vi "createChannel.vi"(8 "error in (no error)":errorcluster, 11 "niDAQmxAO in":refnum<class "niDAQmxAO.lvclass">) -> (0 "error out":errorcluster, 3 "niDAQmxAO out":refnum<class "niDAQmxAO.lvclass">)   [LabVIEW 2009, in "Hardware.lvlib" / "Channels.lvlib" / "niDAQmxAO.lvclass"]
uses:
  niDAQmxAO.lvclass
  <vilib>/DAQmx/create/channels.llb/DAQmx Create Channel (AO-Voltage-Basic).vi
  niDAQmxAO.lvclass/niDAQmxAO.ctl
  <vilib>/DAQmx/create/channels.llb/DAQmx Create Channel (AO-Current-Basic).vi
  <vilib>/DAQmx/create/channels.llb/DAQmx Create Channel (AO-FuncGen).vi
  AnalogOutput.lvclass
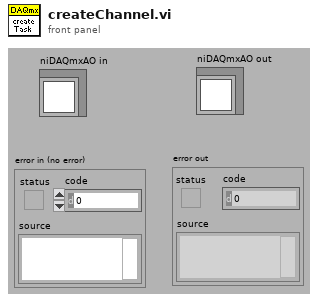
[diagram p1: front panel]
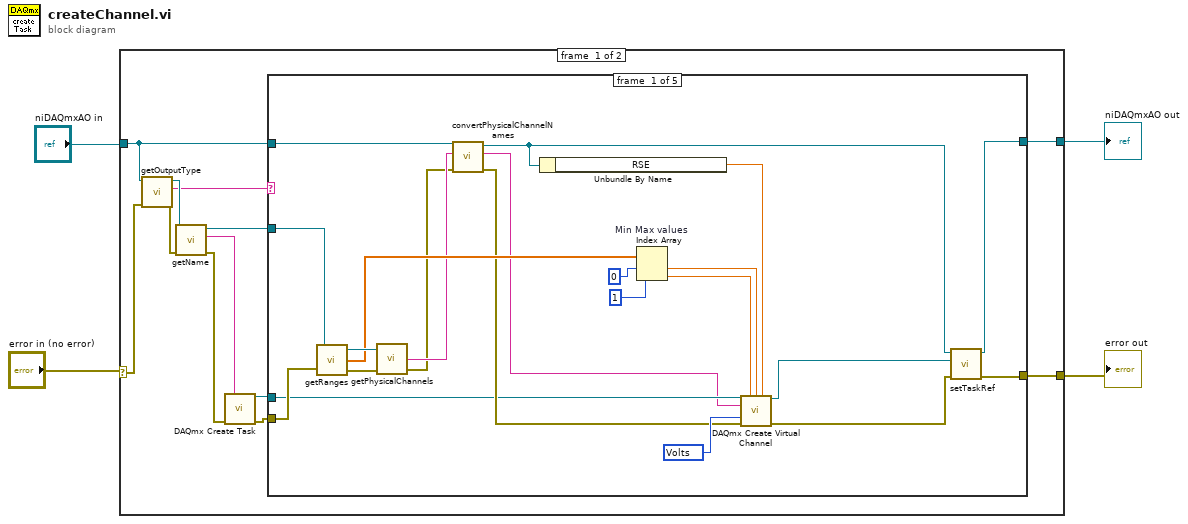
[diagram p0: block diagram]
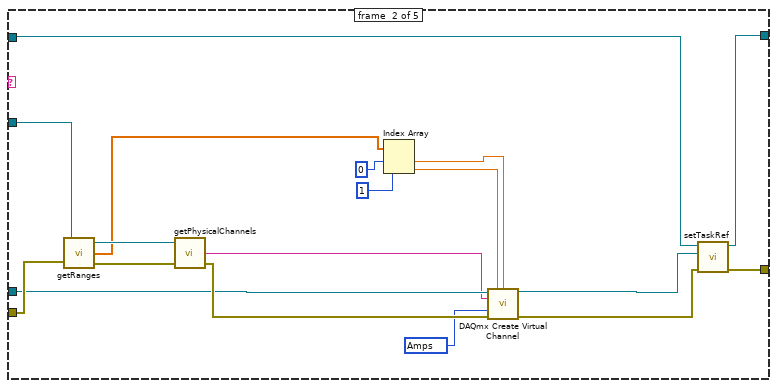
[diagram p2: hidden frame]
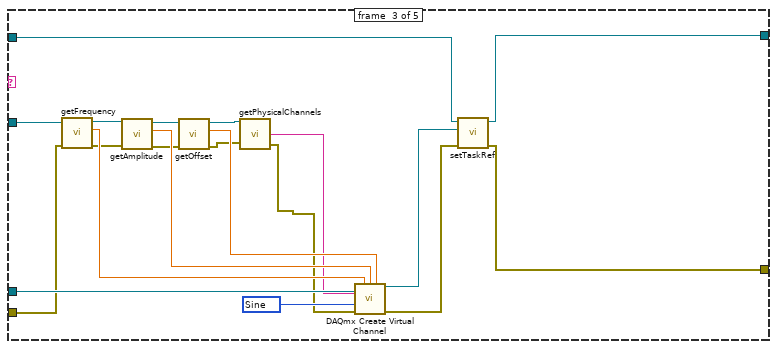
[diagram p3: hidden frame]
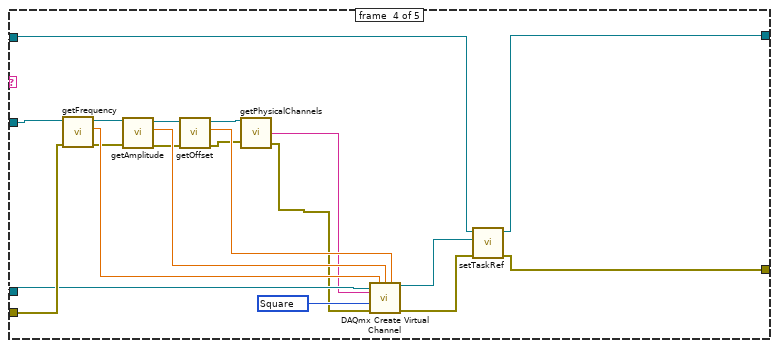
[diagram p4: hidden frame]
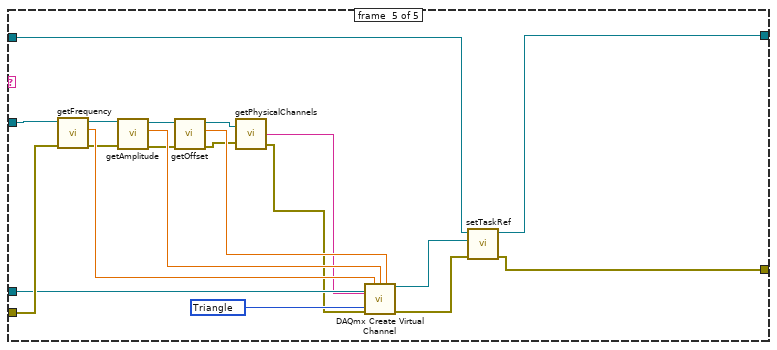
[diagram p5: hidden frame]
diagram:
  n1 = case shown="No Error" "error in (no error)" {
    selector: "error in (no error)" -> [w11 w117]
    tunnel: "niDAQmxAO in" -> [w13 w118]
    tunnel: [w16 w117] -> w2
    tunnel: [w15 w118] -> w1
    frame #0 {
      n2 = call "getOutputType.vi"("error in (no error)"=w11, "AnalogOutput.lvclass in"=w13) -> ("error out"=w10:errorcluster, "Output Type"=w9:string, "AnalogOutput.lvclass out"=w12:refnum<class "niDAQmxAO.lvclass">)  [unwired: 7 in]
      n3 = call "getName.vi"("error in (no error)"=w10, "AnalogOutput.lvclass in"=w12) -> ("error out"=w6:errorcluster, "name"=w5:string, "AnalogOutput.lvclass out"=w14:refnum<class "niDAQmxAO.lvclass">)  [unwired: 7 in]
      n4 = call <vilib>:"DAQmx Create Task.vi"("new task name"=w5, "error in"=w6) -> ("task out"=w8:refnum<k21>, "error out"=w7:errorcluster)  [unwired: 12 in]
      n5 = case shown="\"Voltage\", Default" w9 {
        tunnel: w14 -> [w37 w49 w73 w83 w103]
        tunnel: w8 -> [w18 w47 w62 w81 w101]
        tunnel: w7 -> [w36 w48 w61 w82 w102]
        tunnel: w13 -> [w23 w46 w64 w84 w104]
        tunnel: [w33 w50 w59 w79 w99] -> w16
        tunnel: [w32 w51 w60 w80 w100] -> w15
        frame #0 {
          w25 = u16 10348 items=["Volts"=10348]
          n6 = call "getRanges.vi"("AnalogOutput.lvclass in"=w37, "error in (no error)"=w36) -> ("AnalogOutput.lvclass out"=w31:refnum<class "niDAQmxAO.lvclass">, "Ranges"=w24:dbl[], "error out"=w30:errorcluster)
          n7 = call-dynamic "getPhysicalChannels.vi"("AnalogOutput.lvclass in"=w31, "error in (no error)"=w30) -> ("Physical Channels"=w21:string, "error out"=w20:errorcluster)  [unwired: 1 out]
          n8 = call "convertPhysicalChannelNames.vi"("error in (no error)"=w20, "PhysicalChannels"=w21, "niDAQmxAO.lvclass in"=w23) -> ("error out"=w19:errorcluster, "channel_names"=w17:string, "niDAQmxAO.lvclass out"=w22:refnum<class "niDAQmxAO.lvclass">)  [unwired: 6 in]
          n9 = Unbundle By Name(w22) -> ("RSE"=w38:dbl)
          n10 = Index Array "Min Max values"(array=w24, index #1=0, index #2=1) -> (element #1=w27:dbl, element #2=w26:dbl)
          n11 = call-poly <vilib>:"DAQmx Create Virtual Channel.vi"("task in"=w18, "maximum value"=w26, "minimum value"=w27, "output terminal configuration"=w38, "physical channels"=w17, "units"=w25, "error in"=w19) -> ("task out"=w35:refnum<k21>, "error out"=w34:errorcluster)  [unwired: 7 in]
          n12 = call "setTaskRef.vi"("error in (no error)"=w34, "DAQmx Task Ref"=w35, "niDAQmxAO.lvclass in"=w22) -> ("error out"=w33:errorcluster, "niDAQmxAO.lvclass out"=w32:refnum<class "niDAQmxAO.lvclass">)  [unwired: 7 in]
        }
        frame #1 {
          w43 = u16 10342 items=["Amps"=10342]
          n13 = call "getRanges.vi"("AnalogOutput.lvclass in"=w49, "error in (no error)"=w48) -> ("AnalogOutput.lvclass out"=w54:refnum<class "niDAQmxAO.lvclass">, "Ranges"=w42:dbl[], "error out"=w55:errorcluster)
          n14 = call-dynamic "getPhysicalChannels.vi"("AnalogOutput.lvclass in"=w54, "error in (no error)"=w55) -> ("Physical Channels"=w39:string, "error out"=w56:errorcluster)  [unwired: 1 out]
          n15 = Index Array(array=w42, index #1=0, index #2=1) -> (element #1=w40:dbl, element #2=w41:dbl)
          n16 = call-poly <vilib>:"DAQmx Create Virtual Channel.vi"("task in"=w47, "maximum value"=w41, "minimum value"=w40, "physical channels"=w39, "units"=w43, "error in"=w56) -> ("task out"=w52:refnum<k21>, "error out"=w53:errorcluster)  [unwired: 8 in]
          n17 = call "setTaskRef.vi"("error in (no error)"=w53, "DAQmx Task Ref"=w52, "niDAQmxAO.lvclass in"=w46) -> ("error out"=w50:errorcluster, "niDAQmxAO.lvclass out"=w51:refnum<class "niDAQmxAO.lvclass">)  [unwired: 7 in]
        }
        frame #2 {
          w63 = u16 14751 items=["Sine"=14751]
          n18 = call "getFrequency.vi"("error in (no error)"=w61, "AnalogOutput.lvclass in"=w73) -> ("error out"=w70:errorcluster, "Frequency"=w72:dbl, "AnalogOutput.lvclass out"=w71:refnum<class "niDAQmxAO.lvclass">)  [unwired: 7 in]
          n19 = call "getAmplitude.vi"("error in (no error)"=w70, "AnalogOutput.lvclass in"=w71) -> ("error out"=w68:errorcluster, "Amplitude"=w69:dbl, "AnalogOutput.lvclass out"=w67:refnum<class "niDAQmxAO.lvclass">)  [unwired: 7 in]
          n20 = call "getOffset.vi"("error in (no error)"=w68, "AnalogOutput.lvclass in"=w67) -> ("error out"=w65:errorcluster, "Offset"=w74:dbl, "AnalogOutput.lvclass out"=w66:refnum<class "niDAQmxAO.lvclass">)  [unwired: 7 in]
          n21 = call-dynamic "getPhysicalChannels.vi"("AnalogOutput.lvclass in"=w66, "error in (no error)"=w65) -> ("Physical Channels"=w58:string, "error out"=w57:errorcluster)  [unwired: 1 out]
          n22 = call-poly <vilib>:"DAQmx Create Virtual Channel.vi"("task in"=w62, "frequency"=w72, "amplitude"=w69, "offset"=w74, "physical channels"=w58, "type"=w63, "error in"=w57) -> ("task out"=w75:refnum<k21>, "error out"=w76:errorcluster)  [unwired: 7 in]
          n23 = call "setTaskRef.vi"("error in (no error)"=w76, "DAQmx Task Ref"=w75, "niDAQmxAO.lvclass in"=w64) -> ("error out"=w59:errorcluster, "niDAQmxAO.lvclass out"=w60:refnum<class "niDAQmxAO.lvclass">)  [unwired: 7 in]
        }
        frame #3 {
          w85 = u16 14753 items=["Square"=14753]
          n24 = call "getFrequency.vi"("error in (no error)"=w82, "AnalogOutput.lvclass in"=w83) -> ("error out"=w91:errorcluster, "Frequency"=w93:dbl, "AnalogOutput.lvclass out"=w92:refnum<class "niDAQmxAO.lvclass">)  [unwired: 7 in]
          n25 = call "getAmplitude.vi"("error in (no error)"=w91, "AnalogOutput.lvclass in"=w92) -> ("error out"=w89:errorcluster, "Amplitude"=w90:dbl, "AnalogOutput.lvclass out"=w88:refnum<class "niDAQmxAO.lvclass">)  [unwired: 7 in]
          n26 = call "getOffset.vi"("error in (no error)"=w89, "AnalogOutput.lvclass in"=w88) -> ("error out"=w86:errorcluster, "Offset"=w94:dbl, "AnalogOutput.lvclass out"=w87:refnum<class "niDAQmxAO.lvclass">)  [unwired: 7 in]
          n27 = call-dynamic "getPhysicalChannels.vi"("AnalogOutput.lvclass in"=w87, "error in (no error)"=w86) -> ("Physical Channels"=w78:string, "error out"=w77:errorcluster)  [unwired: 1 out]
          n28 = call-poly <vilib>:"DAQmx Create Virtual Channel.vi"("task in"=w81, "frequency"=w93, "amplitude"=w90, "offset"=w94, "physical channels"=w78, "type"=w85, "error in"=w77) -> ("task out"=w95:refnum<k21>, "error out"=w96:errorcluster)  [unwired: 7 in]
          n29 = call "setTaskRef.vi"("error in (no error)"=w96, "DAQmx Task Ref"=w95, "niDAQmxAO.lvclass in"=w84) -> ("error out"=w79:errorcluster, "niDAQmxAO.lvclass out"=w80:refnum<class "niDAQmxAO.lvclass">)  [unwired: 7 in]
        }
        frame #4 {
          w105 = u16 14752 items=["Triangle"=14752]
          n30 = call "getFrequency.vi"("error in (no error)"=w102, "AnalogOutput.lvclass in"=w103) -> ("error out"=w111:errorcluster, "Frequency"=w113:dbl, "AnalogOutput.lvclass out"=w112:refnum<class "niDAQmxAO.lvclass">)  [unwired: 7 in]
          n31 = call "getAmplitude.vi"("error in (no error)"=w111, "AnalogOutput.lvclass in"=w112) -> ("error out"=w109:errorcluster, "Amplitude"=w110:dbl, "AnalogOutput.lvclass out"=w108:refnum<class "niDAQmxAO.lvclass">)  [unwired: 7 in]
          n32 = call "getOffset.vi"("error in (no error)"=w109, "AnalogOutput.lvclass in"=w108) -> ("error out"=w106:errorcluster, "Offset"=w114:dbl, "AnalogOutput.lvclass out"=w107:refnum<class "niDAQmxAO.lvclass">)  [unwired: 7 in]
          n33 = call-dynamic "getPhysicalChannels.vi"("AnalogOutput.lvclass in"=w107, "error in (no error)"=w106) -> ("Physical Channels"=w98:string, "error out"=w97:errorcluster)  [unwired: 1 out]
          n34 = call-poly <vilib>:"DAQmx Create Virtual Channel.vi"("task in"=w101, "frequency"=w113, "amplitude"=w110, "offset"=w114, "physical channels"=w98, "type"=w105, "error in"=w97) -> ("task out"=w115:refnum<k21>, "error out"=w116:errorcluster)  [unwired: 7 in]
          n35 = call "setTaskRef.vi"("error in (no error)"=w116, "DAQmx Task Ref"=w115, "niDAQmxAO.lvclass in"=w104) -> ("error out"=w99:errorcluster, "niDAQmxAO.lvclass out"=w100:refnum<class "niDAQmxAO.lvclass">)  [unwired: 7 in]
        }
      }
    }
    frame #1 {
    }
  }
  "error out" <- w2
  "niDAQmxAO out" <- w1
